vi "test.vi"() -> ()   [LabVIEW 2018]
uses:
  <vilib>/addons/zeromq/socket_type.ctl
  Socket/Socket.lvclass
  <vilib>/addons/zeromq/socket_options.ctl
  <vilib>/addons/zeromq/zmq_context.lvclass
  <vilib>/addons/zeromq/zeromq.lvlib
panel:
  out "received message":string
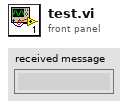
[diagram p1: front panel]
types:
  T1 = typedef "zeromq.lvlib/socket_options.ctl" = enum8{"NONE", "ZMQ_HWM", "<2>", "ZMQ_SWAP", "ZMQ_AFFINITY", "ZMQ_ROUTING_ID", "ZMQ_SUBSCRIBE", "ZMQ_UNSUBSCRIBE", "ZMQ_RATE", "ZMQ_RECOVERY_IVL", "ZMQ_MCAST_LOOP", "ZMQ_SNDBUF", "ZMQ_RCVBUF", "ZMQ_RCVMORE", "ZMQ_FD", "ZMQ_EVENTS", "ZMQ_TYPE", "ZMQ_LINGER", "ZMQ_RECONNECT_IVL", "ZMQ_BACKLOG", "ZMQ_RECOVERY_IVL_MSEC", "ZMQ_RECONNECT_IVL_MAX", "ZMQ_MAXMSGSIZE", "ZMQ_SNDHWM", "ZMQ_RCVHWM", "ZMQ_MULTICAST_HOPS", "<26>", "ZMQ_RCVTIMEO", "ZMQ_SNDTIMEO", "<29>", "<30>", "ZMQ_IPV4ONLY", "ZMQ_LAST_ENDPOINT", "ZMQ_ROUTER_MANDATORY", "ZMQ_TCP_KEEPALIVE", "ZMQ_TCP_KEEPALIVE_CNT", "ZMQ_TCP_KEEPALIVE_IDLE", "ZMQ_TCP_KEEPALIVE_INTVL", "ZMQ_TCP_ACCEPT_FILTER", "ZMQ_IMMEDIATE", "ZMQ_XPUB_VERBOSE", "ZMQ_ROUTER_RAW", "ZMQ_IPV6", "ZMQ_MECHANISM", "ZMQ_PLAIN_SERVER", "ZMQ_PLAIN_USERNAME", "ZMQ_PLAIN_PASSWORD", "ZMQ_CURVE_SERVER", "ZMQ_CURVE_PUBLICKEY", "ZMQ_CURVE_SECRETKEY", "ZMQ_CURVE_SERVERKEY", "ZMQ_PROBE_ROUTER", "ZMQ_REQ_CORRELATE", "ZMQ_REQ_RELAXED", "ZMQ_CONFLATE", "ZMQ_ZAP_DOMAIN", "ZMQ_ROUTER_HANDOVER", "ZMQ_TOS", "ZMQ_IPC_FILTER_PID", "ZMQ_IPC_FILTER_UID", "ZMQ_IPC_FILTER_GID", "ZMQ_CONNECT_ROUTING_ID", "ZMQ_GSSAPI_SERVER", "ZMQ_GSSAPI_PRINCIPAL", "ZMQ_GSSAPI_SERVICE_PRINCIPAL", "ZMQ_GSSAPI_PLAINTEXT", "ZMQ_HANDSHAKE_IVL", "<67>", "ZMQ_SOCKS_PROXY", "ZMQ_XPUB_NODROP", "ZMQ_BLOCKY", "ZMQ_XPUB_MANUAL", "ZMQ_XPUB_WELCOME_MSG", "ZMQ_STREAM_NOTIFY", "ZMQ_INVERT_MATCHING", "ZMQ_HEARTBEAT_IVL", "ZMQ_HEARTBEAT_TTL", "ZMQ_HEARTBEAT_TIMEOUT", "ZMQ_XPUB_VERBOSER", "ZMQ_CONNECT_TIMEOUT", "ZMQ_TCP_MAXRT", "ZMQ_THREAD_SAFE", "<82>", "<83>", "ZMQ_MULTICAST_MAXTPDU", "ZMQ_VMCI_BUFFER_SIZE", "ZMQ_VMCI_BUFFER_MIN_SIZE", "ZMQ_VMCI_BUFFER_MAX_SIZE", "ZMQ_VMCI_CONNECT_TIMEOUT", "ZMQ_USE_FD", "ZMQ_GSSAPI_PRINCIPAL_NAMETYPE", "ZMQ_GSSAPI_SERVICE_PRINCIPAL_NAMETYPE", "ZMQ_BINDTODEVICE", "ZMQ_ZAP_ENFORCE_DOMAIN", "ZMQ_LOOPBACK_FASTPATH", "ZMQ_METADATA", "ZMQ_MULTICAST_LOOP", "ZMQ_ROUTER_NOTIFY"}
  T2 = typedef "zeromq.lvlib/socket_type.ctl" = enum8{"ZMQ_PAIR", "ZMQ_PUB", "ZMQ_SUB", "ZMQ_REQ", "ZMQ_REP", "ZMQ_DEALER", "ZMQ_ROUTER", "ZMQ_PULL", "ZMQ_PUSH", "ZMQ_XPUB", "ZMQ_XSUB", "ZMQ_STREAM", "ZMQ_SERVER", "ZMQ_CLIENT", "ZMQ_RADIO", "ZMQ_DISH", "ZMQ_GATHER", "ZMQ_SCATTER", "ZMQ_DGRAM"}
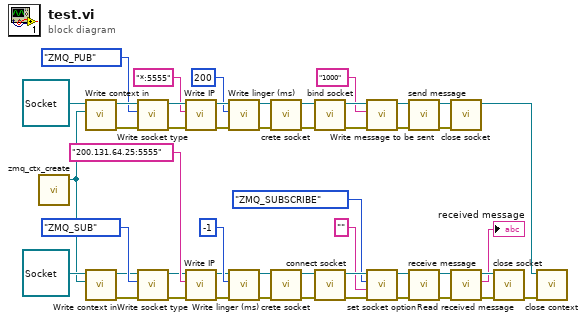
[diagram p0: block diagram]
diagram:
  n1 = call <vilib>:"zmq_ctx_create.vi"() -> ("context out"=w22:refnum<class "zmq_context.lvclass">)  [unwired: 4 in, 1 out]
  n2 = call-dynamic "Write context in.vi"("zeromq.lvlib:ZeroMQ Context"=w22, "Socket in"=refnum<class "Socket.lvclass"> refnum) -> ("error out"=w43:errorcluster, "Socket out"=w48:refnum<class "Socket.lvclass">)  [unwired: 8 in]
  n3 = call-dynamic "Write context in.vi"("zeromq.lvlib:ZeroMQ Context"=w22, "Socket in"=refnum<class "Socket.lvclass"> refnum) -> ("error out"=w29:errorcluster, "Socket out"=w24:refnum<class "Socket.lvclass">)  [unwired: 8 in]
  n4 = call-dynamic "Write socket type.vi"("error in (no error)"=w43, "Socket type"=socket_type."ZMQ_PUB", "Socket in"=w48) -> ("error out"=w44:errorcluster, "Socket out"=w47:refnum<class "Socket.lvclass">)  [unwired: 7 in]
  n5 = call-dynamic "Write socket type.vi"("error in (no error)"=w29, "Socket type"=socket_type."ZMQ_SUB", "Socket in"=w24) -> ("error out"=w28:errorcluster, "Socket out"=w25:refnum<class "Socket.lvclass">)  [unwired: 7 in]
  n6 = call-dynamic "Write IP.vi"("error in (no error)"=w44, "IP"="*:5555", "Socket in"=w47) -> ("error out"=w45:errorcluster, "Socket out"=w46:refnum<class "Socket.lvclass">)  [unwired: 7 in]
  n7 = call-dynamic "Write IP.vi"("error in (no error)"=w28, "IP"="200.131.64.25:5555", "Socket in"=w25) -> ("error out"=w27:errorcluster, "Socket out"=w26:refnum<class "Socket.lvclass">)  [unwired: 7 in]
  n8 = call-dynamic "Write linger (ms).vi"("error in (no error)"=w45, "linger (ms)"=200, "Socket in"=w46) -> ("error out"=w35:errorcluster, "Socket out"=w39:refnum<class "Socket.lvclass">)  [unwired: 7 in]
  n9 = call-dynamic "Write linger (ms).vi"("error in (no error)"=w27, "linger (ms)"=-1, "Socket in"=w26) -> ("error out"=w34:errorcluster, "Socket out"=w33:refnum<class "Socket.lvclass">)  [unwired: 7 in]
  n10 = call "crete socket.vi"("error in (no error)"=w35, "Socket in"=w39) -> ("error out"=w36:errorcluster, "Socket out"=w38:refnum<class "Socket.lvclass">)  [unwired: 8 in]
  n11 = call "crete socket.vi"("error in (no error)"=w34, "Socket in"=w33) -> ("error out"=w20:errorcluster, "Socket out"=w21:refnum<class "Socket.lvclass">)  [unwired: 8 in]
  n12 = call "bind socket.vi"("error in (no error)"=w36, "Socket in"=w38) -> ("error out"=w15:errorcluster, "Socket out"=w14:refnum<class "Socket.lvclass">)  [unwired: 8 in]
  n13 = call "connect socket.vi"("error in (no error)"=w20, "Socket in"=w21) -> ("error out"=w3:errorcluster, "Socket out"=w6:refnum<class "Socket.lvclass">)  [unwired: 8 in]
  n14 = call-dynamic "Write message to be sent.vi"("error in (no error)"=w15, "message to be sent"="1000", "Socket in"=w14) -> ("error out"=w10:errorcluster, "Socket out"=w13:refnum<class "Socket.lvclass">)  [unwired: 7 in]
  n15 = call "set socket option.vi"("error in (no error)"=w3, "value"="" ("message to be sent"), "option"=socket_options."ZMQ_SUBSCRIBE", "Socket2 in"=w6) -> ("error out"=w4:errorcluster, "Socket2 out"=w5:refnum<class "Socket.lvclass">)  [unwired: 6 in]
  n16 = call "send message.vi"("error in (no error)"=w10, "Socket in"=w13) -> ("error out"=w11:errorcluster, "Socket out"=w12:refnum<class "Socket.lvclass">)  [unwired: 8 in]
  n17 = call-dynamic "receive message.vi"("error in (no error)"=w4, "Socket in"=w5) -> ("error out"=w16:errorcluster, "Socket out"=w19:refnum<class "Socket.lvclass">)  [unwired: 8 in]
  n18 = call "close socket.vi"("error in (no error)"=w11, "Socket in"=w12) -> ("Socket out"=w37:refnum<class "Socket.lvclass">)  [unwired: 8 in, 1 out]
  n19 = call-dynamic "Read received message.vi"("error in (no error)"=w16, "Socket in"=w19) -> ("error out"=w17:errorcluster, "received message"=→"received message":string, "Socket out"=w18:refnum<class "Socket.lvclass">)  [unwired: 7 in]
  n20 = call "close socket.vi"("error in (no error)"=w17, "Socket in"=w18) -> ("error out"=w7:errorcluster)  [unwired: 8 in, 1 out]
  n21 = call-dynamic "close context.vi"("error in (no error)"=w7, "Socket in"=w37) -> ()  [unwired: 8 in, 2 out]
